vi "Mass Create Controls.vi"() -> ()   [LabVIEW 2023, in "VILab.lvlib"]
uses:
  VILab.lvlib
  <userlib>/_OpenG.lib/file/file.llb/openg_file.lvlib
  <userlib>/_OpenG.lib/file/file.llb/Convert File Extension (Path)__ogtk.vi
  <vilib>/Utility/traverseref.llb/VI Scripting - Traverse.lvlib
  <vilib>/Utility/traverseref.llb/TRef TravTarget.ctl
panel:
  out "file paths":path[](array[path])
  out "error out":errorcluster
  out "N":i32
  out "i":i32
  in  "error in (no error)":errorcluster
  in  "Decal Root":path
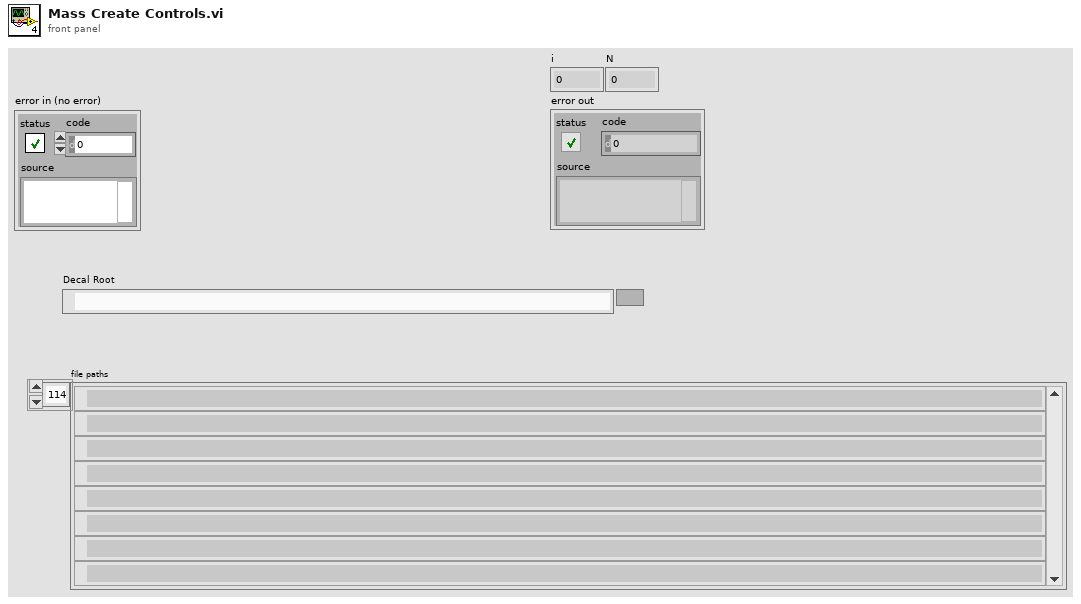
[diagram p1: front panel]
types:
  T1 = typedef "TRef TravTarget.ctl" = enum16{"FP", "BD", "Other"}
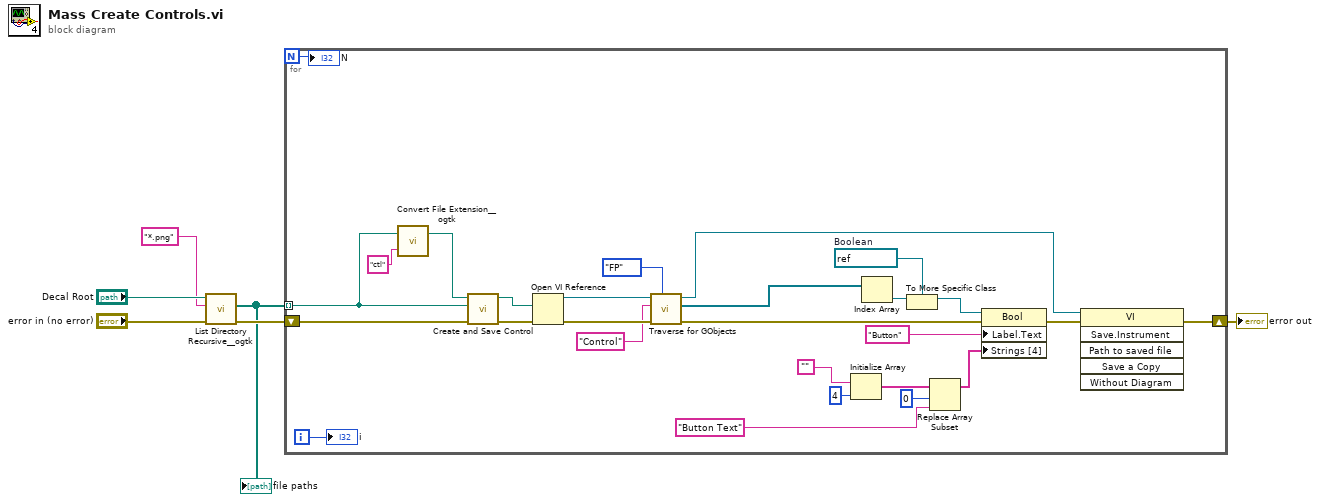
[diagram p0: block diagram]
diagram:
  n1 = call <userlib>:"List Directory Recursive__ogtk.vi"("error in (no error)"="error in (no error)", "pattern"="*.png", "Path"="Decal Root") -> ("error out"=w3:errorcluster, "file paths"=w2:path[])  [unwired: 5 in, 2 out]
  "file paths" <- w2
  n2 = for {
    N -> [w14]
    tunnel: w2 -> [w32] mode=indexing
    shift-right: [w16] -> w1
    shift-left: w3 -> [w33]
    i -> [w15]
    w24 = refnum<vi> refnum  # Boolean
    n3 = call-poly <userlib>:"Convert File Extension__ogtk.vi"("new ending (none)"="ctl", "file name"=w32) -> ("new filename"=w30:path)  [unwired: 1 out]
    n4 = call "Create and Save Control.vi"("error in (no error)"=w33, "PNG Path"=w32, "Save Path"=w30) -> ("error out"=w29:errorcluster, "dup Save Path out"=w28:path)  [unwired: 7 in]
    n5 = Open VI Reference(vi path=w28, error in (no error)=w29) -> (vi reference=w11:refnum<vi>, error out=w12:errorcluster)  [unwired: 4 in]
    n6 = call <vilib>:"Traverse for GObjects.vi"("Traverse Target"=TRef_TravTarget."FP", "error in (no error)"=w12, "Class Name"="Control", "VI Refnum"=w11) -> ("error out"=w7:errorcluster, "References"=w8:refnum<vi>[], "dup VI Refnum"=w9:refnum<vi>)  [unwired: 4 in, 1 out]
    n7 = Initialize Array("", 4 ("dimension size")) -> (w21:string[])
    n8 = Index Array(array=w8) -> (element=w27:refnum<vi>)  [unwired: 1 in]
    n9 = To More Specific Class(target class=w24, reference=w27) -> (specific class reference=w25:refnum<vi>)  [unwired: 1 in, 1 out]
    n10 = Replace Array Subset(array=w21, new element="Button Text" ("Label.Text"), index=0) -> (w18:string[])
    n11 = property class="Bool"(reference=w25, error in=w7, "Label.Text"="Button", "Strings [4]"=w18) -> (error out=w17:errorcluster)  [unwired: 1 out]
    n12 = invoke class="VI" method="Save.Instrument"(reference=w9, error in=w17) -> (error out=w16:errorcluster)  [unwired: 4 in, 5 out]
    "i" <- w15
    "N" <- w14
  }
  "error out" <- w1
